vi "p2.vi"() -> ()   [LabVIEW 2025, in "d5.lvlib"]
uses:
  d5.lvlib
  lv2025-aoc/AOC/AOC.lvlib
panel:
  out "Answer":u64
  in  "Example":string="3-5\n10-14\n16-20\n12-18\n\n1\n5\n8\n11\n17\n32"
  in  "Example 2":bool
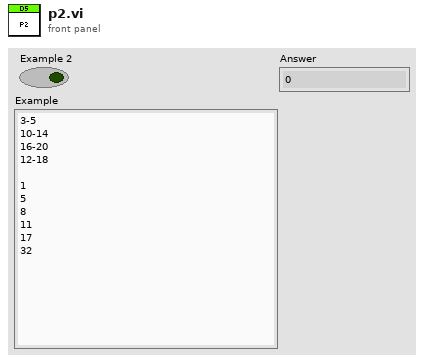
[diagram p1: front panel]
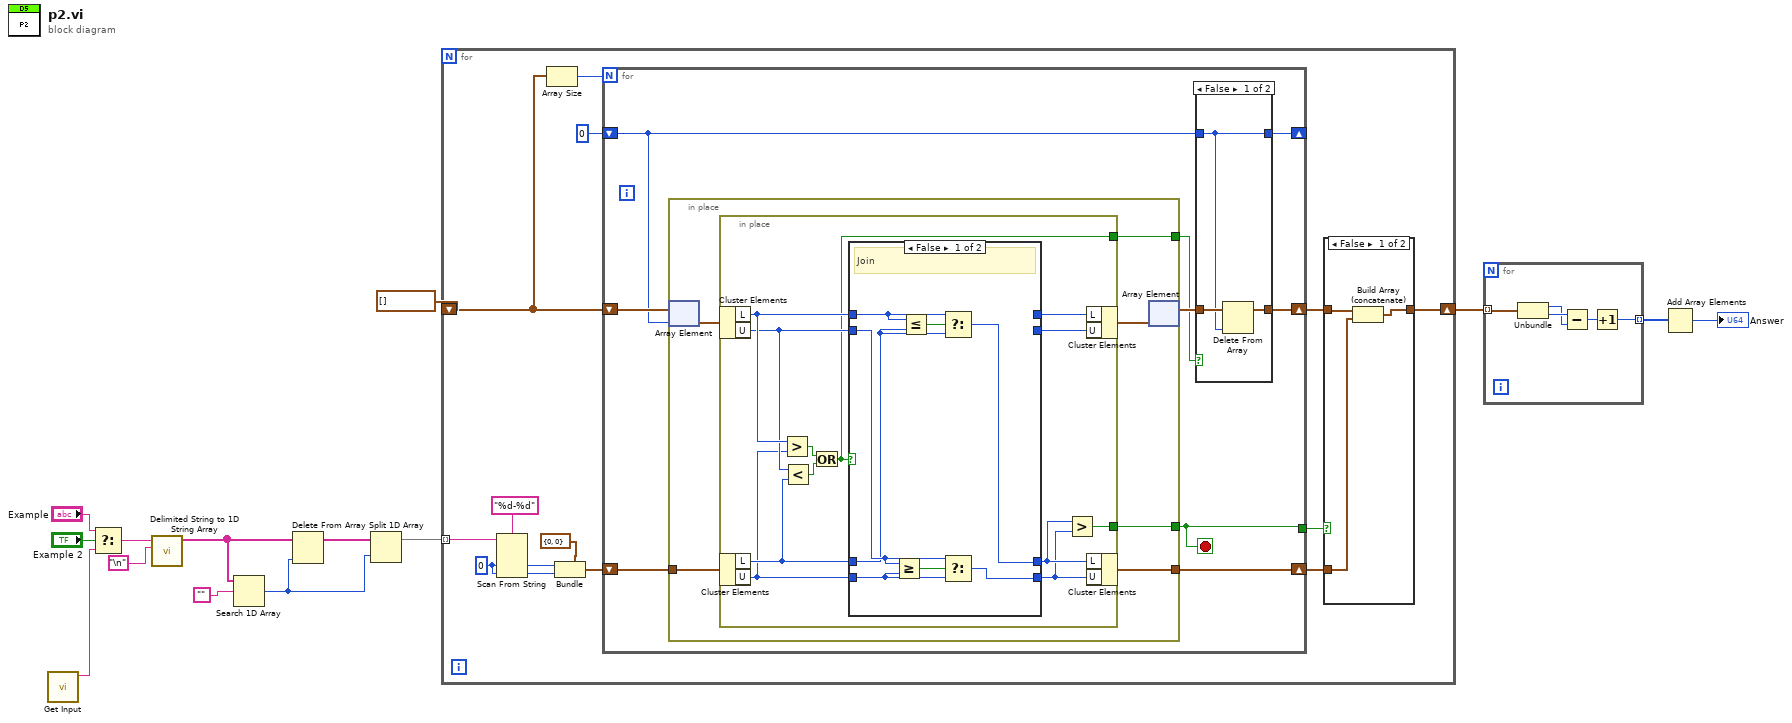
[diagram p0: block diagram]
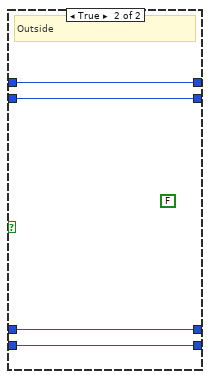
[diagram p2: hidden frame]
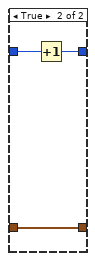
[diagram p3: hidden frame]
diagram:
  n1 = call "Get Input.vi"() -> ("Input"=w12:string)  [unwired: 11 in]
  n2 = Select(t="Example", s="Example 2", f=w12) -> (s? t:f=w11:string)
  n3 = call <vilib>:"Delimited String to 1D String Array.vi"("delimiter"="\n", "delimited string"=w11) -> ("string array"=w7:string[])  [unwired: 9 in]
  n4 = Search 1D Array(1D array=w7, element="") -> (index of element=w5:i32)  [unwired: 1 in]
  n5 = Delete From Array(array=w7, index=w5) -> (array with subset deleted=w6:string[])  [unwired: 1 in, 1 out]
  n6 = Split 1D Array(array=w6, index=w5) -> (first subarray=w4:string[])  [unwired: 1 out]
  n7 = for {
    tunnel: w4 -> [w28] mode=indexing
    shift-right: [w18] -> w2
    shift-left: cluster{"L":u64, "U":u64}[] [] -> [w16]
    w26 = u64 0 ("default value 14")
    n8 = Scan From String(format string="%d-%d", input string=w28, default 1=w26, default 2=w26) -> (output 1=w24:u64, output 2=w23:u64)  [unwired: 2 in, 3 out]
    n9 = Array Size(array=w16) -> (size(s)=w25:i32)
    n10 = Bundle(cluster=cluster{"L":u64, "U":u64} {"L"=0, "U"=0} ("Cluster"), "L"=w24, "U"=w23) -> (w22:cluster{"L":u64, "U":u64})
    n11 = for {
      N: w25 -> [_]
      shift-right: [w32] -> w19
      shift-left: w16 -> [w37]
      shift-right: [w35] -> w20
      shift-left: w22 -> [w36]
      tunnel: [w34] -> w21
      shift-right: [w31] -> _
      shift-left: 0 -> [w30]
      stop <- w34 stop-if-true
      n12 = in-place {
        in-place-border: w36 -> [w41]
        in-place-border: [w40] -> w35
        in-place-border: [w39] -> w34
        in-place-border: [w38] -> w29
        n13 = in-place-array #1(w37, w30) -> (w43:cluster{"L":u64, "U":u64})
        n14 = in-place {
          in-place-border: [w45] -> w39
          in-place-border: [w44] -> w38
          n15 = in-place-cluster #2(w43) -> ("L"=w55:u64, "U"=w52:u64)
          n16 = in-place-cluster #3(w41) -> ("L"=w49:u64, "U"=w48:u64)
          n17 = Greater?(x=w55, y=w48) -> (0:w50:bool)
          n18 = Less?(x=w52, y=w49) -> (x < y?=w51:bool)
          n19 = Or(x=w50, y=w51) -> (x .or. y?=w44:bool)
          n20 = case shown="False" w44 {
            tunnel: w55 -> [w59 w67]
            tunnel: [_ w67] -> w54
            tunnel: [_ w66] -> w53
            tunnel: w52 -> [w62 w66]
            tunnel: w49 -> [w61 w65]
            tunnel: [w56 w65] -> w47
            tunnel: [w57 w64] -> w46
            tunnel: w48 -> [w58 w64]
            frame False {
              # "Join"
              n21 = Greater Or Equal?(x=w62, y=w58) -> (x >= y?=w60:bool)
              n22 = Less Or Equal?(x=w59, y=w61) -> (x <= y?=w63:bool)
              n23 = Select(t=w59, s=w63, f=w61) -> (s? t:f=w56:u64)
              n24 = Select(t=w62, s=w60, f=w58) -> (s? t:f=w57:u64)
            }
            frame True {
              (unwired) FALSE
              # "Outside"
            }
          }
          n25 = Greater?(x=w47, y=w46) -> (0:w45:bool)
          n26 = in-place-cluster #2("L"=w54, "U"=w53) -> (w42:cluster{"L":u64, "U":u64})
          n27 = in-place-cluster #3("L"=w47, "U"=w46) -> (w40:cluster{"L":u64, "U":u64})
        }
        n28 = in-place-array #1(w42) -> (w33:cluster{"L":u64, "U":u64}[])  [unwired: 1 out]
      }
      n29 = case shown="False" w29 {
        tunnel: w33 -> [w70 w73]
        tunnel: [w69 w73] -> w32
        tunnel: w30 -> [w68 w72]
        tunnel: [w68 w71] -> w31
        frame False {
          n30 = Delete From Array(array=w70, index=w68) -> (array with subset deleted=w69:cluster{"L":u64, "U":u64}[])  [unwired: 1 in, 1 out]
        }
        frame True {
          n31 = Increment(x=w72) -> (x+1=w71:i32)
        }
      }
    }
    n32 = case shown="False" w21 {
      tunnel: w20 -> [w75 _]
      tunnel: w19 -> [w76 w77]
      tunnel: [w74 w77] -> w18
      frame False {
        n33 = Build Array (concatenate)(w76, w75) -> (w74:cluster{"L":u64, "U":u64}[])
      }
      frame True {
      }
    }
  }
  n34 = for {
    tunnel: w2 -> [w82] mode=indexing
    tunnel: [w78] -> w1 mode=indexing
    n35 = Unbundle(w82) -> ("L"=w80:u64, "U"=w81:u64)
    n36 = Subtract(x=w81, y=w80) -> (x-y=w79:u64)
    n37 = Increment(x=w79) -> (x+1=w78:u64)
  }
  n38 = Add Array Elements(numeric array=w1) -> (sum=→"Answer":u64)
